vi "Optiscan.vi"(4 "Parameter in":dbl[](array[numeric]), 5 "error in (no error)":errorcluster, 6 "Timeout":u32=100, 7 "VISA resource name":refnum<visa-resource-name>, 8 "Command":T1(ring)) -> (0 "error out":errorcluster, 2 "Status out":bool[](array[boolean]), 3 "Parameter out":dbl[](array[numeric]))   [LabVIEW 2015]
uses:
  <vilib>/Instr/_visa.llb/VISA Open Access Mode.ctl
  <vilib>/Instr/_visa.llb/VISA Configure Serial Port (Instr).vi
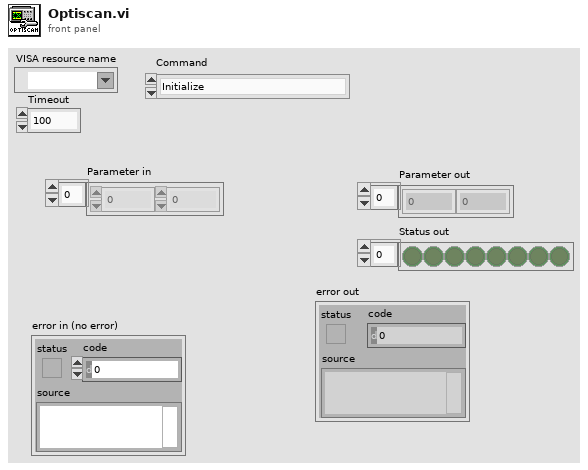
[diagram p1: front panel]
types:
  T1 = enum16{"Initialize", "Close", "Move Absolute", "Get Position", "Move Relative", "Set Acceleration", "Get Acceleration", "Set Speed", "Get Speed", "Limit Switch Status", "Motor Status", "Stop (controlled)", "Stop (instant)"}
  T2 = typedef "VISA Open Access Mode.ctl" = u32
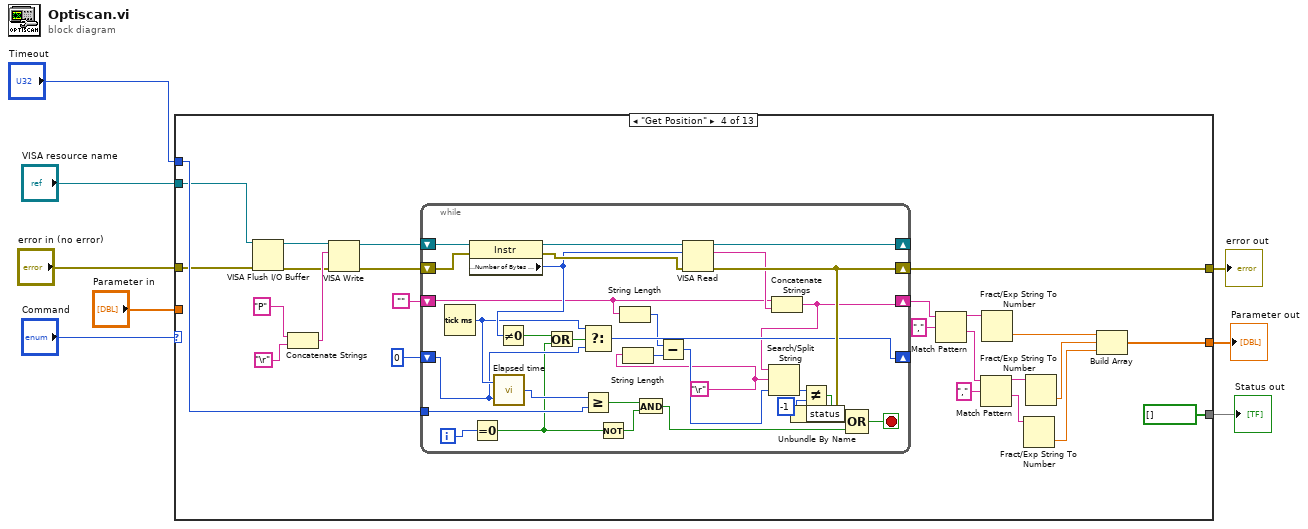
[diagram p0: block diagram]
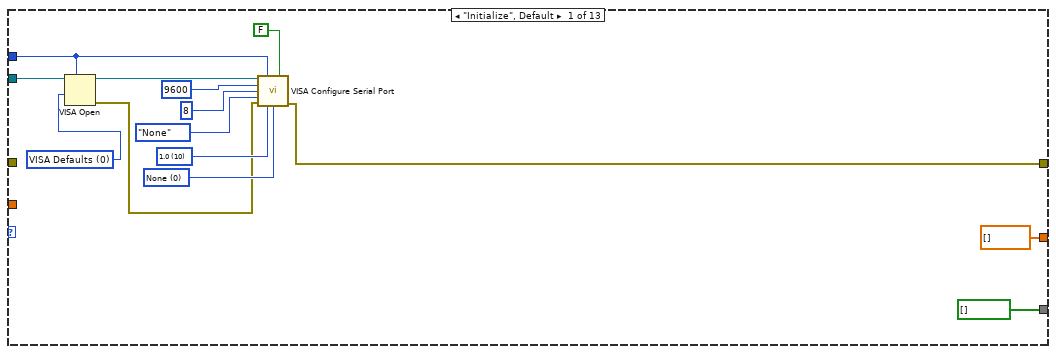
[diagram p2: hidden frame]
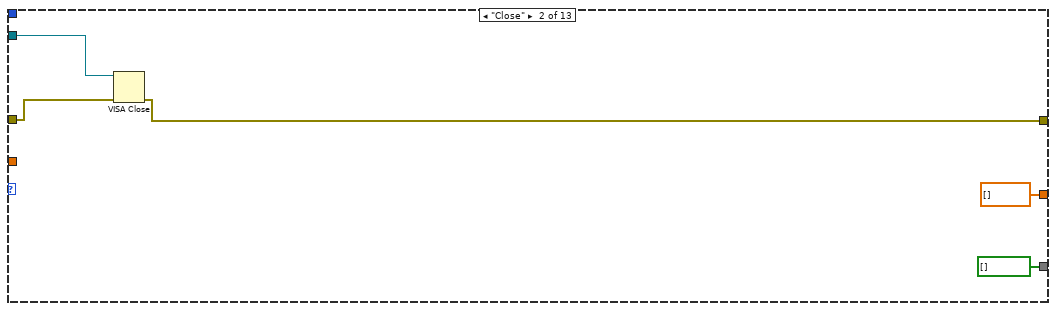
[diagram p3: hidden frame]
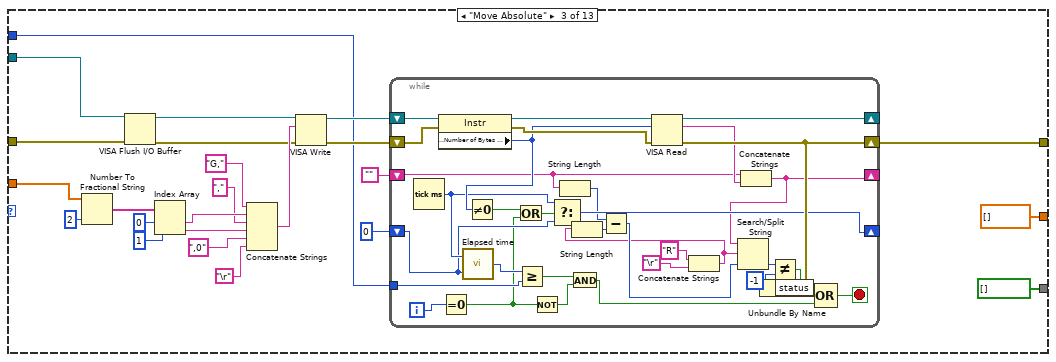
[diagram p4: hidden frame]
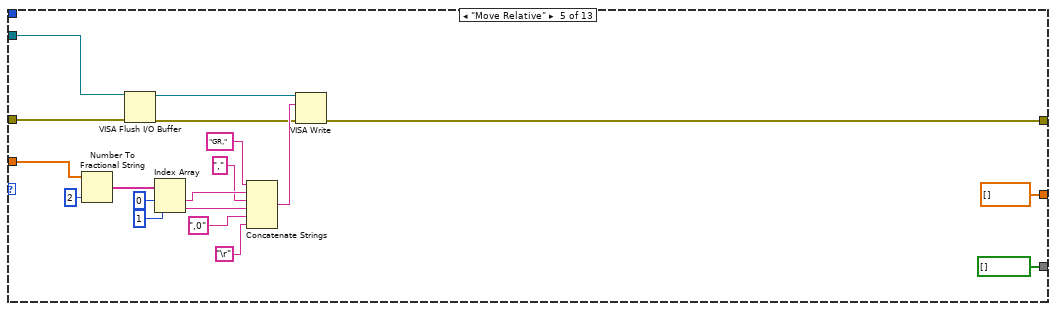
[diagram p5: hidden frame]
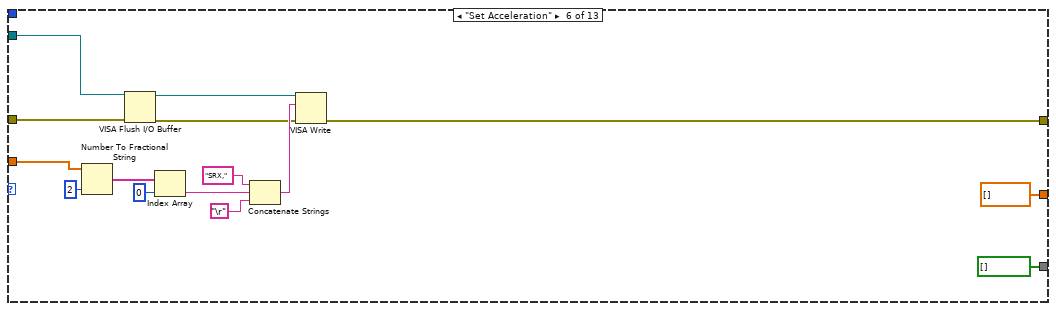
[diagram p6: hidden frame]
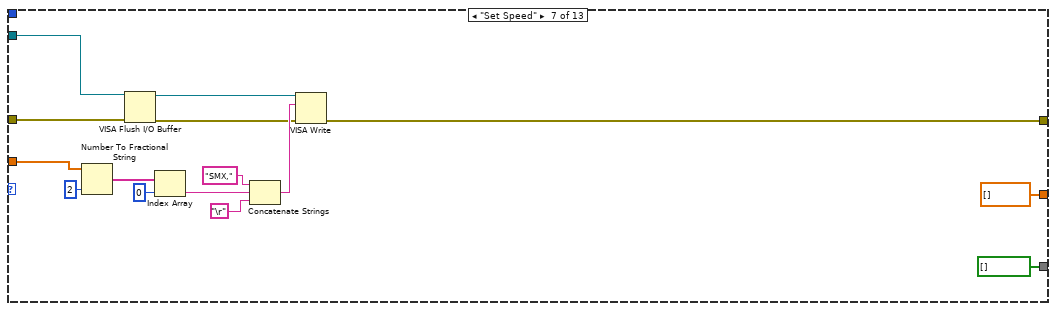
[diagram p7: hidden frame]
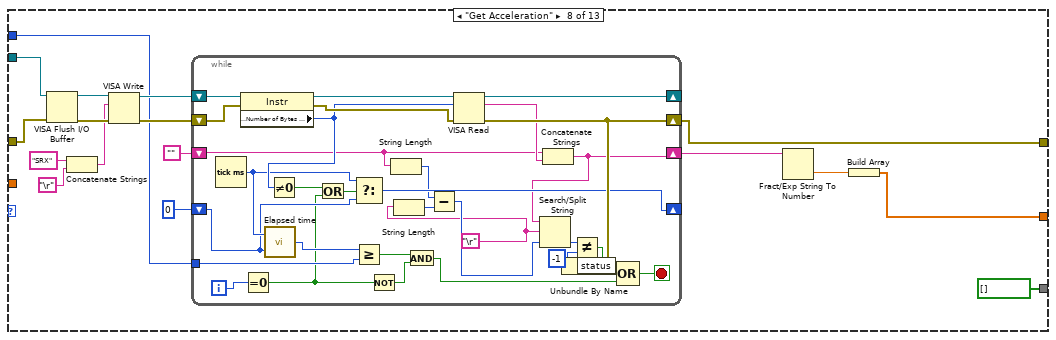
[diagram p8: hidden frame]
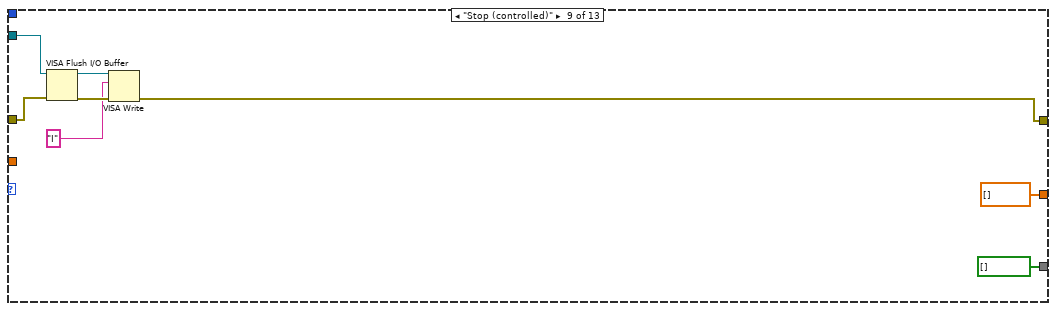
[diagram p9: hidden frame]
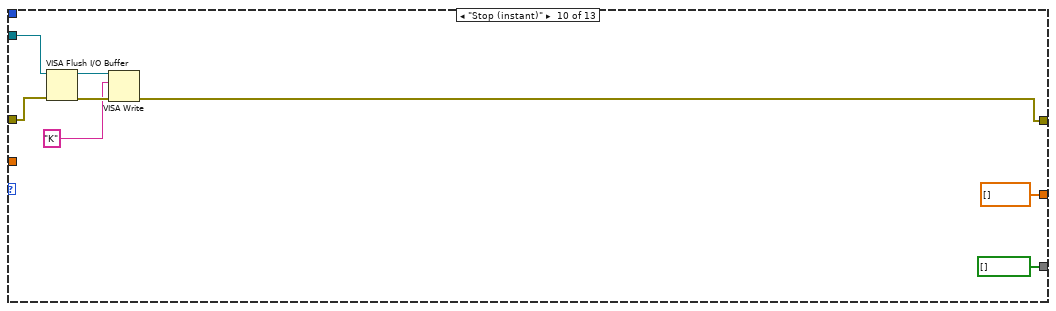
[diagram p10: hidden frame]
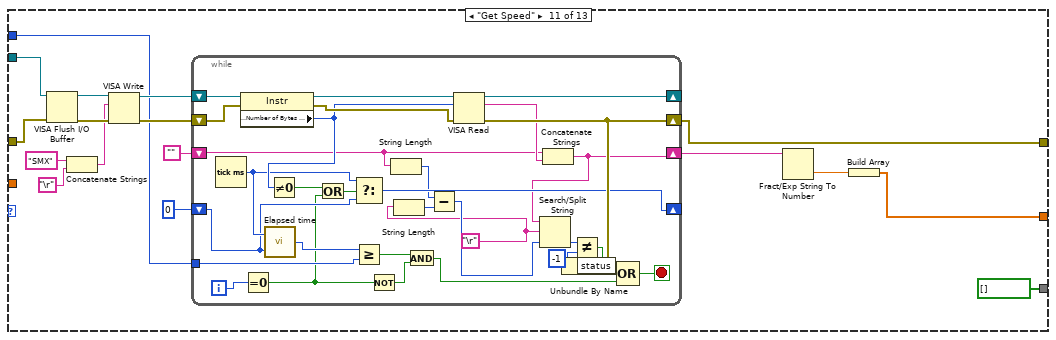
[diagram p11: hidden frame]
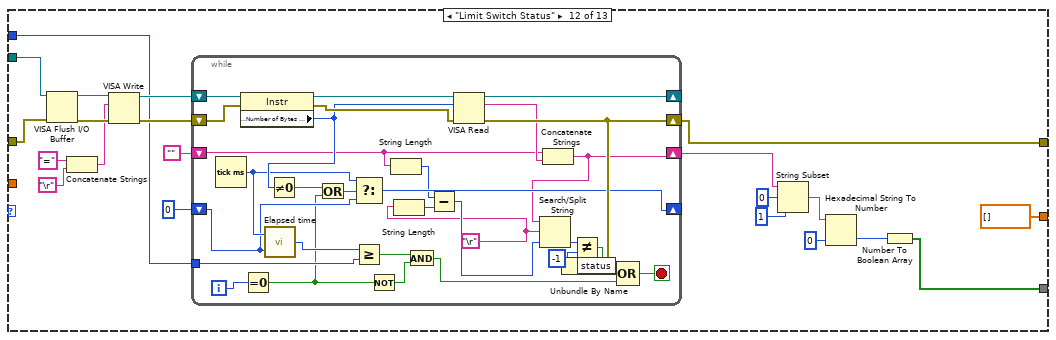
[diagram p12: hidden frame]
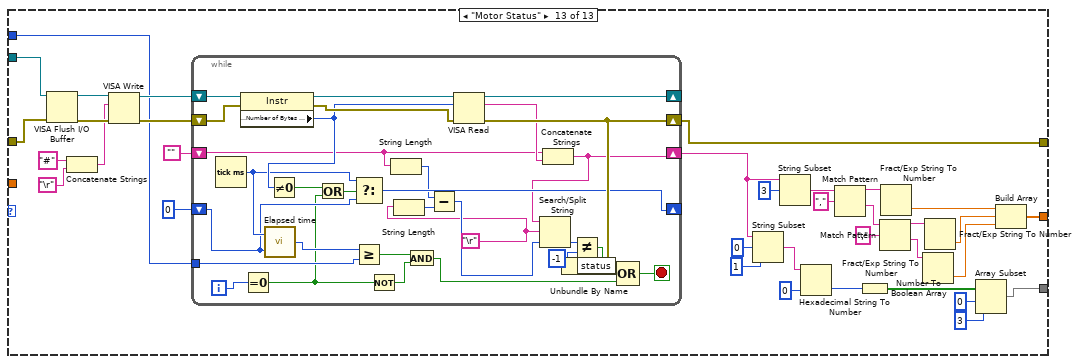
[diagram p13: hidden frame]
diagram:
  n1 = case shown="\"Get Position\"" "Command" {
    tunnel: [w11 w25 w28 w101 w154 w169 w184 w193 w240 w248 w257 w310 w376] -> w8
    tunnel: "Timeout" -> [w14 _ w29 w100 _ _ _ w195 _ _ w259 w311 w377]
    tunnel: "VISA resource name" -> [w16 w27 w48 w99 w156 w171 w186 w204 w243 w251 w268 w320 w386]
    tunnel: "error in (no error)" -> [_ w26 w47 w98 w155 w170 w185 w203 w242 w250 w267 w319 w385]
    tunnel: "Parameter in" -> [_ _ w43 _ w150 w165 w180 _ _ _ _ _ _]
    tunnel: [dbl[] [] dbl[] [] dbl[] [] w88 dbl[] [] dbl[] [] dbl[] [] w191 dbl[] [] dbl[] [] w255 dbl[] [] w361] -> w2
    tunnel: [bool[] [] ("Array") bool[] [] ("Array") bool[] [] ("Array") bool[] [] ("Array") bool[] [] ("Array") bool[] [] ("Array") bool[] [] ("Array") bool[] [] ("Array") bool[] [] ("Array") bool[] [] ("Array") bool[] [] ("Array") w303 w357] -> w1
    frame "Initialize", Default {
      w13 = T2 0 items=["VISA Defaults"=0, "Exclusive Lock"=1, "Load Configured Settings"=4] ("Access Mode")
      w17 = u16 0 items=["None", "XON/XOFF", "RTS/CTS", "XON/XOFF & RTS/CTS", "DTR/DSR", "XON/XOFF & DTR/DSR"] ("flow control (0:none)")
      w18 = u16 10 items=["1.0"=10, "1.5"=15, "2.0"=20] ("stop bits (10: 1 bit)")
      n2 = VISA Open(timeout (0)=w14, access mode=w13, VISA resource name=w16) -> (VISA resource name=w15:refnum<visa-resource-name>, error out=w12:errorcluster)  [unwired: 2 in]
      n3 = call-poly "VISA Configure Serial Port"("VISA resource name"=w15, "timeout (10sec)"=w14, "Enable Termination\nChar (T)"=FALSE ("Enable Termination\nChar (T)"), "baud rate (9600)"=u32 9600, "data bits (8)"=u16 8, "parity (0:none)"=enum16{"None", "Odd", "Even", "Mark", "Space"}."None", "error in (no error)"=w12, "stop bits (10: 1 bit)"=w18, "flow control (0:none)"=w17) -> ("error out"=w11:errorcluster)  [unwired: 5 in, 1 out]
    }
    frame "Close" {
      n4 = VISA Close(VISA resource name=w27, error in (no error)=w26) -> (error out=w25:errorcluster)
    }
    frame "Move Absolute" {
      n5 = Number To Fractional String(number=w43, precision (6)=i16 2) -> (F-format string=w44:string[])  [unwired: 2 in]
      n6 = VISA Flush I/O Buffer(VISA resource name=w48, error in (no error)=w47) -> (VISA resource name out=w51:refnum<visa-resource-name>, error out=w49:errorcluster)  [unwired: 1 in]
      n7 = Index Array(array=w44, index #1=0 ("index"), index #2=1 ("index")) -> (element #1=w41:string, element #2=w37:string)
      n8 = Concatenate Strings("G,", w41, "," ("string"), w37, ",0" ("string"), "\r") -> (w50:string)
      n9 = VISA Write(VISA resource name=w51, write buffer=w50, error in (no error)=w49) -> (VISA resource name out=w30:refnum<visa-resource-name>, error out=w31:errorcluster)  [unwired: 1 out]
      n10 = while {
        shift-right: [w80] -> _
        shift-left: w30 -> [w84]
        shift-right: [w78] -> w28
        shift-left: w31 -> [w83]
        shift-right: [w60] -> _
        shift-left: "" -> [w59]
        shift-right: [w68] -> _
        shift-left: u32 0 -> [w65]
        tunnel: w29 -> [w66]
        i -> [w71]
        stop <- w79 stop-if-true
        n11 = Tick Count (ms)() -> (millisecond timer value=w69:u32)
        n12 = property class="Instr"(reference=w84, error in=w83) -> (reference out=w82:refnum<visa-resource-name>, error out=w81:errorcluster, "Serial Settings:Number of Bytes at Serial Port"=w73:u32)
        n13 = Equal To 0?(x=w71) -> (x = 0?=w61:bool)
        n14 = call "Elapsed time.vi"("Start time (ms)"=w65, "Current time (ms)"=w69) -> ("Elapsed time"=w67:u32)
        n15 = Not Equal To 0?(x=w73) -> (x != 0?=w72:bool)
        n16 = Or(x=w72, y=w61) -> (x .or. y?=w70:bool)
        n17 = Greater Or Equal?(x=w67, y=w66) -> (x >= y?=w63:bool)
        n18 = Not(x=w61) -> (.not. x?=w62:bool)
        n19 = Select(t=w69, s=w70, f=w65) -> (s? t:f=w68:u32)
        n20 = String Length(string=w59) -> (length=w57:i32)
        n21 = And(x=w63, y=w62) -> (x .and. y?=w64:bool)
        n22 = VISA Read(VISA resource name=w82, byte count=w73, error in (no error)=w81) -> (VISA resource name out=w80:refnum<visa-resource-name>, read buffer=w77:string, error out=w78:errorcluster)  [unwired: 1 out]
        n23 = Concatenate Strings("R" ("string"), "\r") -> (w54:string)
        n24 = String Length(string=w54) -> (length=w58:i32)
        n25 = Subtract(x=w57, y=w58) -> (x-y=w56:i32)
        n26 = Concatenate Strings(w59, w77) -> (w60:string)
        n27 = Search/Split String(string=w60, search string/char (-)=w54, offset (0)=w56) -> (offset of match=w76:i32)  [unwired: 2 out]
        n28 = Unbundle By Name(w78) -> ("status"=w53:bool)
        n29 = Not Equal?(x=w76, y=-1) -> (x != y?=w74:bool)
        n30 = Compound Arithmetic op=OR(w53, w74, w64) -> (w79:bool)
      }
    }
    frame "Get Position" {
      n31 = VISA Flush I/O Buffer(VISA resource name=w99, error in (no error)=w98) -> (VISA resource name out=w108:refnum<visa-resource-name>, error out=w106:errorcluster)  [unwired: 1 in]
      n32 = Concatenate Strings("P", "\r") -> (w107:string)
      n33 = VISA Write(VISA resource name=w108, write buffer=w107, error in (no error)=w106) -> (VISA resource name out=w105:refnum<visa-resource-name>, error out=w104:errorcluster)  [unwired: 1 out]
      n34 = while {
        shift-right: [w136] -> _
        shift-left: w105 -> [w140]
        shift-right: [w134] -> w101
        shift-left: w104 -> [w139]
        shift-right: [w116] -> w96
        shift-left: "" -> [w115]
        shift-right: [w124] -> _
        shift-left: u32 0 -> [w121]
        tunnel: w100 -> [w122]
        i -> [w127]
        stop <- w135 stop-if-true
        w110 = "\r"
        n35 = Tick Count (ms)() -> (millisecond timer value=w125:u32)
        n36 = property class="Instr"(reference=w140, error in=w139) -> (reference out=w138:refnum<visa-resource-name>, error out=w137:errorcluster, "Serial Settings:Number of Bytes at Serial Port"=w129:u32)
        n37 = Equal To 0?(x=w127) -> (x = 0?=w117:bool)
        n38 = call "Elapsed time.vi"("Start time (ms)"=w121, "Current time (ms)"=w125) -> ("Elapsed time"=w123:u32)
        n39 = Not Equal To 0?(x=w129) -> (x != 0?=w128:bool)
        n40 = Or(x=w128, y=w117) -> (x .or. y?=w126:bool)
        n41 = Select(t=w125, s=w126, f=w121) -> (s? t:f=w124:u32)
        n42 = Greater Or Equal?(x=w123, y=w122) -> (x >= y?=w119:bool)
        n43 = Not(x=w117) -> (.not. x?=w118:bool)
        n44 = String Length(string=w115) -> (length=w113:i32)
        n45 = String Length(string=w110) -> (length=w114:i32)
        n46 = And(x=w119, y=w118) -> (x .and. y?=w120:bool)
        n47 = Subtract(x=w113, y=w114) -> (x-y=w112:i32)
        n48 = VISA Read(VISA resource name=w138, byte count=w129, error in (no error)=w137) -> (VISA resource name out=w136:refnum<visa-resource-name>, read buffer=w133:string, error out=w134:errorcluster)  [unwired: 1 out]
        n49 = Concatenate Strings(w115, w133) -> (w116:string)
        n50 = Search/Split String(string=w116, search string/char (-)=w110, offset (0)=w112) -> (offset of match=w132:i32)  [unwired: 2 out]
        n51 = Unbundle By Name(w134) -> ("status"=w111:bool)
        n52 = Not Equal?(x=w132, y=-1) -> (x != y?=w130:bool)
        n53 = Compound Arithmetic op=OR(w111, w130, w120) -> (w135:bool)
      }
      n54 = Match Pattern(string=w96, regular expression=",") -> (before substring=w93:string, after substring=w91:string)  [unwired: 1 in, 2 out]
      n55 = Match Pattern(string=w91, regular expression=",") -> (before substring=w90:string, after substring=w89:string)  [unwired: 1 in, 2 out]
      n56 = Fract/Exp String To Number(string=w93) -> (number=w94:dbl)  [unwired: 3 in, 1 out]
      n57 = Fract/Exp String To Number(string=w89) -> (number=w86:dbl)  [unwired: 3 in, 1 out]
      n58 = Fract/Exp String To Number(string=w90) -> (number=w87:dbl)  [unwired: 3 in, 1 out]
      n59 = Build Array(w94, w87, w86) -> (w88:dbl[])
    }
    frame "Move Relative" {
      n60 = Number To Fractional String(number=w150, precision (6)=i16 2) -> (F-format string=w151:string[])  [unwired: 2 in]
      n61 = VISA Flush I/O Buffer(VISA resource name=w156, error in (no error)=w155) -> (VISA resource name out=w159:refnum<visa-resource-name>, error out=w157:errorcluster)  [unwired: 1 in]
      n62 = Index Array(array=w151, index #1=0 ("index"), index #2=1 ("index")) -> (element #1=w148:string, element #2=w144:string)
      n63 = Concatenate Strings("GR,", w148, "," ("string"), w144, ",0" ("string"), "\r") -> (w158:string)
      n64 = VISA Write(VISA resource name=w159, write buffer=w158, error in (no error)=w157) -> (error out=w154:errorcluster)  [unwired: 2 out]
    }
    frame "Set Acceleration" {
      n65 = Number To Fractional String(number=w165, precision (6)=i16 2) -> (F-format string=w166:string[])  [unwired: 2 in]
      n66 = VISA Flush I/O Buffer(VISA resource name=w171, error in (no error)=w170) -> (VISA resource name out=w174:refnum<visa-resource-name>, error out=w172:errorcluster)  [unwired: 1 in]
      n67 = Index Array(array=w166, index=0) -> (element=w163:string)
      n68 = Concatenate Strings("SRX,", w163, "\r") -> (w173:string)
      n69 = VISA Write(VISA resource name=w174, write buffer=w173, error in (no error)=w172) -> (error out=w169:errorcluster)  [unwired: 2 out]
    }
    frame "Set Speed" {
      n70 = Number To Fractional String(number=w180, precision (6)=i16 2) -> (F-format string=w181:string[])  [unwired: 2 in]
      n71 = VISA Flush I/O Buffer(VISA resource name=w186, error in (no error)=w185) -> (VISA resource name out=w189:refnum<visa-resource-name>, error out=w187:errorcluster)  [unwired: 1 in]
      n72 = Index Array(array=w181, index=0) -> (element=w178:string)
      n73 = Concatenate Strings("SMX,", w178, "\r") -> (w188:string)
      n74 = VISA Write(VISA resource name=w189, write buffer=w188, error in (no error)=w187) -> (error out=w184:errorcluster)  [unwired: 2 out]
    }
    frame "Get Acceleration" {
      n75 = VISA Flush I/O Buffer(VISA resource name=w204, error in (no error)=w203) -> (VISA resource name out=w206:refnum<visa-resource-name>, error out=w205:errorcluster)  [unwired: 1 in]
      n76 = Concatenate Strings("SRX" ("string"), "\r") -> (w202:string)
      n77 = VISA Write(VISA resource name=w206, write buffer=w202, error in (no error)=w205) -> (VISA resource name out=w196:refnum<visa-resource-name>, error out=w197:errorcluster)  [unwired: 1 out]
      n78 = while {
        shift-right: [w233] -> _
        shift-left: w196 -> [w237]
        shift-right: [w231] -> w193
        shift-left: w197 -> [w236]
        shift-right: [w213] -> w194
        shift-left: "" -> [w212]
        shift-right: [w221] -> _
        shift-left: u32 0 -> [w218]
        tunnel: w195 -> [w219]
        i -> [w224]
        stop <- w232 stop-if-true
        w207 = "\r"
        n79 = Tick Count (ms)() -> (millisecond timer value=w222:u32)
        n80 = property class="Instr"(reference=w237, error in=w236) -> (reference out=w235:refnum<visa-resource-name>, error out=w234:errorcluster, "Serial Settings:Number of Bytes at Serial Port"=w226:u32)
        n81 = Equal To 0?(x=w224) -> (x = 0?=w214:bool)
        n82 = call "Elapsed time.vi"("Start time (ms)"=w218, "Current time (ms)"=w222) -> ("Elapsed time"=w220:u32)
        n83 = Not Equal To 0?(x=w226) -> (x != 0?=w225:bool)
        n84 = Or(x=w225, y=w214) -> (x .or. y?=w223:bool)
        n85 = Select(t=w222, s=w223, f=w218) -> (s? t:f=w221:u32)
        n86 = Greater Or Equal?(x=w220, y=w219) -> (x >= y?=w216:bool)
        n87 = Not(x=w214) -> (.not. x?=w215:bool)
        n88 = String Length(string=w212) -> (length=w210:i32)
        n89 = String Length(string=w207) -> (length=w211:i32)
        n90 = And(x=w216, y=w215) -> (x .and. y?=w217:bool)
        n91 = Subtract(x=w210, y=w211) -> (x-y=w209:i32)
        n92 = VISA Read(VISA resource name=w235, byte count=w226, error in (no error)=w234) -> (VISA resource name out=w233:refnum<visa-resource-name>, read buffer=w230:string, error out=w231:errorcluster)  [unwired: 1 out]
        n93 = Concatenate Strings(w212, w230) -> (w213:string)
        n94 = Search/Split String(string=w213, search string/char (-)=w207, offset (0)=w209) -> (offset of match=w229:i32)  [unwired: 2 out]
        n95 = Unbundle By Name(w231) -> ("status"=w208:bool)
        n96 = Not Equal?(x=w229, y=-1) -> (x != y?=w227:bool)
        n97 = Compound Arithmetic op=OR(w208, w227, w217) -> (w232:bool)
      }
      n98 = Fract/Exp String To Number(string=w194) -> (number=w192:dbl)  [unwired: 3 in, 1 out]
      n99 = Build Array(w192) -> (w191:dbl[])
    }
    frame "Stop (controlled)" {
      n100 = VISA Flush I/O Buffer(VISA resource name=w243, error in (no error)=w242) -> (VISA resource name out=w245:refnum<visa-resource-name>, error out=w244:errorcluster)  [unwired: 1 in]
      n101 = VISA Write(VISA resource name=w245, write buffer="I" ("string"), error in (no error)=w244) -> (error out=w240:errorcluster)  [unwired: 2 out]
    }
    frame "Stop (instant)" {
      n102 = VISA Flush I/O Buffer(VISA resource name=w251, error in (no error)=w250) -> (VISA resource name out=w253:refnum<visa-resource-name>, error out=w252:errorcluster)  [unwired: 1 in]
      n103 = VISA Write(VISA resource name=w253, write buffer="K" ("string"), error in (no error)=w252) -> (error out=w248:errorcluster)  [unwired: 2 out]
    }
    frame "Get Speed" {
      n104 = VISA Flush I/O Buffer(VISA resource name=w268, error in (no error)=w267) -> (VISA resource name out=w270:refnum<visa-resource-name>, error out=w269:errorcluster)  [unwired: 1 in]
      n105 = Concatenate Strings("SMX" ("string"), "\r") -> (w266:string)
      n106 = VISA Write(VISA resource name=w270, write buffer=w266, error in (no error)=w269) -> (VISA resource name out=w260:refnum<visa-resource-name>, error out=w261:errorcluster)  [unwired: 1 out]
      n107 = while {
        shift-right: [w297] -> _
        shift-left: w260 -> [w301]
        shift-right: [w295] -> w257
        shift-left: w261 -> [w300]
        shift-right: [w277] -> w258
        shift-left: "" -> [w276]
        shift-right: [w285] -> _
        shift-left: u32 0 -> [w282]
        tunnel: w259 -> [w283]
        i -> [w288]
        stop <- w296 stop-if-true
        w271 = "\r"
        n108 = Tick Count (ms)() -> (millisecond timer value=w286:u32)
        n109 = property class="Instr"(reference=w301, error in=w300) -> (reference out=w299:refnum<visa-resource-name>, error out=w298:errorcluster, "Serial Settings:Number of Bytes at Serial Port"=w290:u32)
        n110 = Equal To 0?(x=w288) -> (x = 0?=w278:bool)
        n111 = call "Elapsed time.vi"("Start time (ms)"=w282, "Current time (ms)"=w286) -> ("Elapsed time"=w284:u32)
        n112 = Not Equal To 0?(x=w290) -> (x != 0?=w289:bool)
        n113 = Or(x=w289, y=w278) -> (x .or. y?=w287:bool)
        n114 = Select(t=w286, s=w287, f=w282) -> (s? t:f=w285:u32)
        n115 = Greater Or Equal?(x=w284, y=w283) -> (x >= y?=w280:bool)
        n116 = Not(x=w278) -> (.not. x?=w279:bool)
        n117 = String Length(string=w276) -> (length=w274:i32)
        n118 = String Length(string=w271) -> (length=w275:i32)
        n119 = And(x=w280, y=w279) -> (x .and. y?=w281:bool)
        n120 = Subtract(x=w274, y=w275) -> (x-y=w273:i32)
        n121 = VISA Read(VISA resource name=w299, byte count=w290, error in (no error)=w298) -> (VISA resource name out=w297:refnum<visa-resource-name>, read buffer=w294:string, error out=w295:errorcluster)  [unwired: 1 out]
        n122 = Concatenate Strings(w276, w294) -> (w277:string)
        n123 = Search/Split String(string=w277, search string/char (-)=w271, offset (0)=w273) -> (offset of match=w293:i32)  [unwired: 2 out]
        n124 = Unbundle By Name(w295) -> ("status"=w272:bool)
        n125 = Not Equal?(x=w293, y=-1) -> (x != y?=w291:bool)
        n126 = Compound Arithmetic op=OR(w272, w291, w281) -> (w296:bool)
      }
      n127 = Fract/Exp String To Number(string=w258) -> (number=w256:dbl)  [unwired: 3 in, 1 out]
      n128 = Build Array(w256) -> (w255:dbl[])
    }
    frame "Limit Switch Status" {
      n129 = VISA Flush I/O Buffer(VISA resource name=w320, error in (no error)=w319) -> (VISA resource name out=w322:refnum<visa-resource-name>, error out=w321:errorcluster)  [unwired: 1 in]
      n130 = Concatenate Strings("=" ("string"), "\r") -> (w318:string)
      n131 = VISA Write(VISA resource name=w322, write buffer=w318, error in (no error)=w321) -> (VISA resource name out=w312:refnum<visa-resource-name>, error out=w313:errorcluster)  [unwired: 1 out]
      n132 = while {
        shift-right: [w349] -> _
        shift-left: w312 -> [w353]
        shift-right: [w347] -> w310
        shift-left: w313 -> [w352]
        shift-right: [w329] -> w309
        shift-left: "" -> [w328]
        shift-right: [w337] -> _
        shift-left: u32 0 -> [w334]
        tunnel: w311 -> [w335]
        i -> [w340]
        stop <- w348 stop-if-true
        w323 = "\r"
        n133 = Tick Count (ms)() -> (millisecond timer value=w338:u32)
        n134 = property class="Instr"(reference=w353, error in=w352) -> (reference out=w351:refnum<visa-resource-name>, error out=w350:errorcluster, "Serial Settings:Number of Bytes at Serial Port"=w342:u32)
        n135 = Equal To 0?(x=w340) -> (x = 0?=w330:bool)
        n136 = call "Elapsed time.vi"("Start time (ms)"=w334, "Current time (ms)"=w338) -> ("Elapsed time"=w336:u32)
        n137 = Not Equal To 0?(x=w342) -> (x != 0?=w341:bool)
        n138 = Or(x=w341, y=w330) -> (x .or. y?=w339:bool)
        n139 = Select(t=w338, s=w339, f=w334) -> (s? t:f=w337:u32)
        n140 = Greater Or Equal?(x=w336, y=w335) -> (x >= y?=w332:bool)
        n141 = Not(x=w330) -> (.not. x?=w331:bool)
        n142 = String Length(string=w328) -> (length=w326:i32)
        n143 = String Length(string=w323) -> (length=w327:i32)
        n144 = And(x=w332, y=w331) -> (x .and. y?=w333:bool)
        n145 = Subtract(x=w326, y=w327) -> (x-y=w325:i32)
        n146 = VISA Read(VISA resource name=w351, byte count=w342, error in (no error)=w350) -> (VISA resource name out=w349:refnum<visa-resource-name>, read buffer=w346:string, error out=w347:errorcluster)  [unwired: 1 out]
        n147 = Concatenate Strings(w328, w346) -> (w329:string)
        n148 = Search/Split String(string=w329, search string/char (-)=w323, offset (0)=w325) -> (offset of match=w345:i32)  [unwired: 2 out]
        n149 = Unbundle By Name(w347) -> ("status"=w324:bool)
        n150 = Not Equal?(x=w345, y=-1) -> (x != y?=w343:bool)
        n151 = Compound Arithmetic op=OR(w324, w343, w333) -> (w348:bool)
      }
      n152 = String Subset(string=w309, offset (0)=0, length (rest)=1 ("length (rest)")) -> (substring=w306:string)
      n153 = Hexadecimal String To Number(string=w306, default (0uL)=u16 0 ("default (0 U32)")) -> (number=w304:u16)  [unwired: 1 in, 1 out]
      n154 = Number To Boolean Array(number=w304) -> (Boolean array=w303:bool[])
    }
    frame "Motor Status" {
      n155 = VISA Flush I/O Buffer(VISA resource name=w386, error in (no error)=w385) -> (VISA resource name out=w388:refnum<visa-resource-name>, error out=w387:errorcluster)  [unwired: 1 in]
      n156 = Concatenate Strings("#" ("string"), "\r") -> (w384:string)
      n157 = VISA Write(VISA resource name=w388, write buffer=w384, error in (no error)=w387) -> (VISA resource name out=w378:refnum<visa-resource-name>, error out=w379:errorcluster)  [unwired: 1 out]
      n158 = while {
        shift-right: [w415] -> _
        shift-left: w378 -> [w419]
        shift-right: [w413] -> w376
        shift-left: w379 -> [w418]
        shift-right: [w395] -> w360
        shift-left: "" -> [w394]
        shift-right: [w403] -> _
        shift-left: u32 0 -> [w400]
        tunnel: w377 -> [w401]
        i -> [w406]
        stop <- w414 stop-if-true
        w389 = "\r"
        n159 = Tick Count (ms)() -> (millisecond timer value=w404:u32)
        n160 = property class="Instr"(reference=w419, error in=w418) -> (reference out=w417:refnum<visa-resource-name>, error out=w416:errorcluster, "Serial Settings:Number of Bytes at Serial Port"=w408:u32)
        n161 = Equal To 0?(x=w406) -> (x = 0?=w396:bool)
        n162 = call "Elapsed time.vi"("Start time (ms)"=w400, "Current time (ms)"=w404) -> ("Elapsed time"=w402:u32)
        n163 = Not Equal To 0?(x=w408) -> (x != 0?=w407:bool)
        n164 = Or(x=w407, y=w396) -> (x .or. y?=w405:bool)
        n165 = Select(t=w404, s=w405, f=w400) -> (s? t:f=w403:u32)
        n166 = Greater Or Equal?(x=w402, y=w401) -> (x >= y?=w398:bool)
        n167 = Not(x=w396) -> (.not. x?=w397:bool)
        n168 = String Length(string=w394) -> (length=w392:i32)
        n169 = String Length(string=w389) -> (length=w393:i32)
        n170 = And(x=w398, y=w397) -> (x .and. y?=w399:bool)
        n171 = Subtract(x=w392, y=w393) -> (x-y=w391:i32)
        n172 = VISA Read(VISA resource name=w417, byte count=w408, error in (no error)=w416) -> (VISA resource name out=w415:refnum<visa-resource-name>, read buffer=w412:string, error out=w413:errorcluster)  [unwired: 1 out]
        n173 = Concatenate Strings(w394, w412) -> (w395:string)
        n174 = Search/Split String(string=w395, search string/char (-)=w389, offset (0)=w391) -> (offset of match=w411:i32)  [unwired: 2 out]
        n175 = Unbundle By Name(w413) -> ("status"=w390:bool)
        n176 = Not Equal?(x=w411, y=-1) -> (x != y?=w409:bool)
        n177 = Compound Arithmetic op=OR(w390, w409, w399) -> (w414:bool)
      }
      n178 = String Subset(string=w360, offset (0)=0, length (rest)=1 ("length (rest)")) -> (substring=w373:string)
      n179 = String Subset(string=w360, offset (0)=3) -> (substring=w359:string)  [unwired: 1 in]
      n180 = Hexadecimal String To Number(string=w373, default (0uL)=u16 0 ("default (0 U32)")) -> (number=w371:u16)  [unwired: 1 in, 1 out]
      n181 = Match Pattern(string=w359, regular expression=",") -> (before substring=w368:string, after substring=w366:string)  [unwired: 1 in, 2 out]
      n182 = Number To Boolean Array(number=w371) -> (Boolean array=w356:bool[])
      n183 = Match Pattern(string=w366, regular expression=",") -> (before substring=w365:string, after substring=w364:string)  [unwired: 1 in, 2 out]
      n184 = Fract/Exp String To Number(string=w368) -> (number=w369:dbl)  [unwired: 3 in, 1 out]
      n185 = Fract/Exp String To Number(string=w364) -> (number=w362:dbl)  [unwired: 3 in, 1 out]
      n186 = Fract/Exp String To Number(string=w365) -> (number=w363:dbl)  [unwired: 3 in, 1 out]
      n187 = Array Subset(array=w356, index=0, length=3) -> (w357:bool[])
      n188 = Build Array(w369, w363, w362) -> (w361:dbl[])
    }
  }
  "error out" <- w8
  "Parameter out" <- w2
  "Status out" <- w1
